vi "Set Down Sampling Threshold.vi"(8 "error in (no error)":errorcluster, 10 "Value":dbl, 11 "BarcodeDetector in":refnum<class "BarcodeDetector.lvclass">) -> (0 "error out":errorcluster, 3 "BarcodeDetector (Duplicate)":refnum<class "BarcodeDetector.lvclass">)   [LabVIEW 2020, in "g_ar_toolkit.feature_detection.lvlib" / "BarcodeDetector.lvclass"]
uses:
  BarcodeDetector.lvclass
  BarcodeDetector.lvclass/BarcodeDetector.ctl
  g_ar_toolkit.common/Module Path.vi
  <vilib>/Utility/error.llb/Error Cluster From Error Code.vi
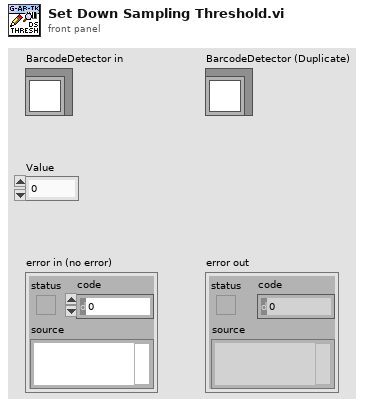
[diagram p1: front panel]
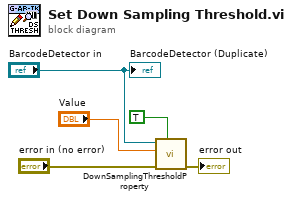
[diagram p0: block diagram]
diagram:
  n1 = call "DownSamplingThresholdProperty.vi"("Write?"=TRUE, "error in (no error)"="error in (no error)", "Value in"="Value", "BarcodeDetector in"="BarcodeDetector in") -> ("error out"=→"error out":errorcluster)  [unwired: 6 in, 1 out]
  "BarcodeDetector (Duplicate)" <- "BarcodeDetector in"
